vi "Read shift.vi"(11 "Node in":refnum<class "INode.lvclass">) -> (2 "shift":i64, 3 "Node out":refnum<class "INode.lvclass">)   [LabVIEW 2021, in "d20.lvlib" / "INode.lvclass"]
uses:
  INode.lvclass
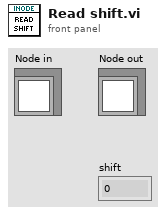
[diagram p1: front panel]
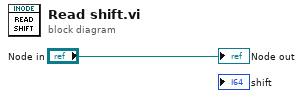
[diagram p0: block diagram]
diagram:
  "Node out" <- "Node in"
